vi "SR430.read data.vi"(0 "i ref in":refnum<vi>, 5 "error in (no error)":errorcluster) -> (14 "i ref out":refnum<vi>, 16 "Output Waveform":T1, 19 "error out":errorcluster)   [LabVIEW 2014, in "SR430.lvlib"]
doc: "gets the data in binary format from the SR430. The data format is a waveform flattened to string.\n\nThis method performs a sequence of the following methods.\n\n- stop scan\n- read bin data\n- clear records\n- start scan"
uses:
  SR430.lvlib
  CS_Core/CSSystem/CoreDefs/CoreDefs.rawDataType.ctl
  CS_Core/CSApplicationBaseClasses/MCSBase/MCSBase.statusType.ctl
  CS_Core/CSApplicationBaseClasses/MCSBase/MCSBase.directionType.ctl
  CS_Core/CSApplicationBaseClasses/MCSBase/MCSBase.serviceType.ctl
  CSlibraries/UtilityLib/UtilityLib.valueStatus.ctl
  CS_Core/CSApplicationBaseClasses/MCSBase/MCSBase.lvlib
  CSlibraries/UtilityLib/UtilityLib.lvlib
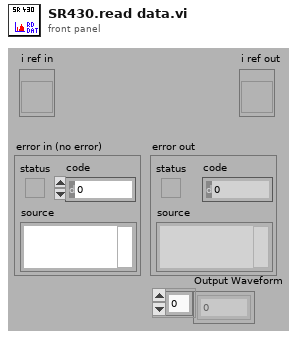
[diagram p1: front panel]
types:
  T1 = typedef "CoreDefs.rawDataType.ctl" = i8[]
  T2 = typedef "UtilityLib.lvlib/UtilityLib.valueStatus.ctl" = enum16{"no info available", "stand by/off", "on", "warning", "alarm/malfunction", "not implemented", "user action required", "important information", "system default", "control default", "indicator default", "button default"}
  T3 = typedef "MCSBase.lvlib/MCSBase.serviceType.ctl" = enum16{"counts", "totalCounts", "binWidth", "nOfBins", "nOfRecords", "status", "discrLevel", "discrSlope", "triggerLevel", "triggerSlope"}
  T4 = typedef "MCSBase.lvlib/MCSBase.directionType.ctl" = enum16{"unknown", "update actual value", "update nominal value", "update both"}
  T5 = typedef "MCSBase.lvlib/MCSBase.statusType.ctl" = i32
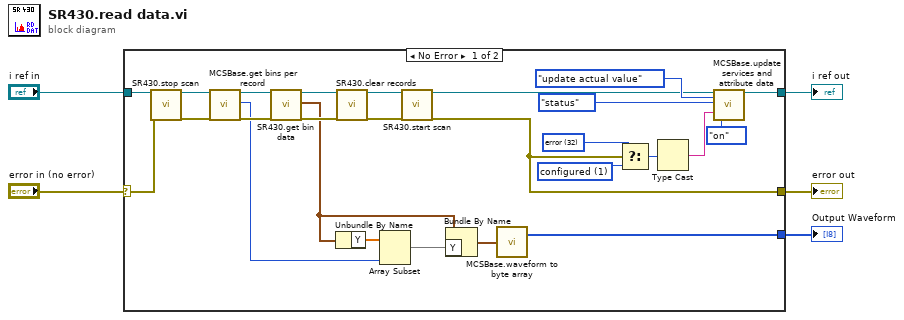
[diagram p0: block diagram]
diagram:
  n1 = case shown="No Error" "error in (no error)" {
    selector: "error in (no error)" -> [w19 w32]
    tunnel: "i ref in" -> [w31 w33]
    tunnel: [w7 w32] -> w4
    tunnel: [w8 w33] -> w3
    tunnel: [w17 _] -> w2
    frame No Error {
      w13 = T5 32 items=["unknown"=0, "configured"=1, "error"=32] ("t")
      w12 = T5 1 items=["unknown"=0, "configured"=1, "error"=32] ("service")
      n2 = call "SR430.stop scan.vi"("i ref in"=w31, "error in (no error)"=w19) -> ("i ref out"=w24:refnum<vi>, "error out"=w23:errorcluster)  [unwired: 16 in]
      n3 = call "MCSBase.get bins per record.vi"("i ref in"=w24, "error in (no error)"=w23) -> ("i ref out"=w26:refnum<vi>, "nOfBins"=w6:i32, "error out"=w25:errorcluster)  [unwired: 15 in]
      n4 = call "SR430.get bin data.vi"("i ref in"=w26, "error in (no error)"=w25) -> ("i ref out"=w30:refnum<vi>, "Output Waveform"=w20:waveform(dbl), "error out"=w29:errorcluster)  [unwired: 15 in]
      n5 = Unbundle By Name(w20) -> ("Y"=w22:dbl[])
      n6 = call "SR430.clear records.vi"("i ref in"=w30, "error in (no error)"=w29) -> ("i ref out"=w28:refnum<vi>, "error out"=w27:errorcluster)  [unwired: 16 in]
      n7 = Array Subset(array=w22, length=w6) -> (w21:dbl[])  [unwired: 1 in]
      n8 = call "SR430.start scan.vi"("i ref in"=w28, "error in (no error)"=w27) -> ("i ref out"=w9:refnum<vi>, "error out"=w7:errorcluster)  [unwired: 16 in]
      n9 = Bundle By Name(cluster=w20, "Y"=w21) -> (w18:waveform(dbl))
      n10 = call "MCSBase.waveform to byte array.vi"("Waveform"=w18) -> ("byteArray out"=w17:T1)  [unwired: 1 out]
      n11 = Select(t=w13, s=w7, f=w12) -> (s? t:f=w14:T5)
      n12 = Type Cast(x=w14) -> (*(type *) &x=w15:string)  [unwired: 1 in]
      n13 = call "MCSBase.update services and attribute data.vi"("i ref in"=w9, "direction"=MCSBase.directionType."update actual value", "service"=MCSBase.serviceType."status", "value"=w15, "quality"=UtilityLib.valueStatus."on") -> ("i ref out"=w8:refnum<vi>)  [unwired: 12 in, 2 out]
    }
    frame Error {
    }
  }
  "error out" <- w4
  "i ref out" <- w3
  "Output Waveform" <- w2
